vi "initializeRobotModelTest.vi"(4 "V_sample":dbl, 5 "start":bool, 6 "delta":dbl, 7 "V_sent":dbl, 9 "Samples":dbl, 11 "fixed_V_sent?":bool=TRUE) -> (1 "RobotModelAllInformation out":T1={"distance"=0.0, "lastRobotPosition"=[], "timestampOn2ndStateStart"=timestamp(0 s since 1904-01-01), "sampleCount"=0, "stateInMachine"=0, "crashCases"=[], "lastEstVel"=inf, "IdealVelocities"=[], "RealVelocities"=[], "testFinished?"=FALSE, "RobotModelArray"=[]}, 2 "totalNumberOfTests":dbl, 3 "triples (V0, Vf, V_sent)":dbl[][](array[numeric])=[[-6.5, -7.0, -7.0, 0.0], [-6.0, -7.0, -7.0, 1.0], [-5.5, -7.0, -7.0, 2.0], [-5.0, -7.0, -7.0, 3.0], [-4.5, -7.0, -7.0, 4.0], [-4.0, -7.0, -7.0, 5.0], [-3.5, -7.0, -7.0, 6.0], [-3.0, -7.0, -7.0, 7.0], [-2.5, -7.0, -7.0, 8.0], [-2.0, -7.0, -7.0, 9.0], [-1.5, -7.0, -7.0, 10.0], [-1.0, -7.0, -7.0, 11.0], [-0.5, -7.0, -7.0, 12.0], [0.0, -7.0, -7.0, 13.0], [-7.0, -6.5, -6.5, 14.0], [-6.0, -6.5, -6.5, 15.0], [-5.5, -6.5, -6.5, 16.0], [-5.0, -6.5, -6.5, 17.0], [-4.5, -6.5, -6.5, 18.0], [-4.0, -6.5, -6.5, 19.0], [-3.5, -6.5, -6.5, 20.0], [-3.0, -6.5, -6.5, 21.0], [-2.5, -6.5, -6.5, 22.0], [-2.0, -6.5, -6.5, 23.0], [-1.5, -6.5, -6.5, 24.0], [-1.0, -6.5, -6.5, 25.0], [-0.5, -6.5, -6.5, 26.0], [0.0, -6.5, -6.5, 27.0], [-7.0, -6.0, -6.0, 28.0], [-6.5, -6.0, -6.0, 29.0], [-5.5, -6.0, -6.0, 30.0], [-5.0, -6.0, -6.0, 31.0], [-4.5, -6.0, -6.0, 32.0], [-4.0, -6.0, -6.0, 33.0], [-3.5, -6.0, -6.0, 34.0], [-3.0, -6.0, -6.0, 35.0], [-2.5, -6.0, -6.0, 36.0], [-2.0, -6.0, -6.0, 37.0], [-1.5, -6.0, -6.0, 38.0], [-1.0, -6.0, -6.0, 39.0], [-0.5, -6.0, -6.0, 40.0], [0.0, -6.0, -6.0, 41.0], [-7.0, -5.5, -5.5, 42.0], [-6.5, -5.5, -5.5, 43.0], [-6.0, -5.5, -5.5, 44.0], [-5.0, -5.5, -5.5, 45.0], [-4.5, -5.5, -5.5, 46.0], [-4.0, -5.5, -5.5, 47.0], [-3.5, -5.5, -5.5, 48.0], [-3.0, -5.5, -5.5, 49.0], [-2.5, -5.5, -5.5, 50.0], [-2.0, -5.5, -5.5, 51.0], [-1.5, -5.5, -5.5, 52.0], [-1.0, -5.5, -5.5, 53.0], [-0.5, -5.5, -5.5, 54.0], [0.0, -5.5, -5.5, 55.0], [-7.0, -5.0, -5.0, 56.0], [-6.5, -5.0, -5.0, 57.0], [-6.0, -5.0, -5.0, 58.0], [-5.5, -5.0, -5.0, 59.0], [-4.5, -5.0, -5.0, 60.0], [-4.0, -5.0, -5.0, 61.0], [-3.5, -5.0, -5.0, 62.0], [-3.0, -5.0, -5.0, 63.0], [-2.5, -5.0, -5.0, 64.0], [-2.0, -5.0, -5.0, 65.0], [-1.5, -5.0, -5.0, 66.0], [-1.0, -5.0, -5.0, 67.0], [-0.5, -5.0, -5.0, 68.0], [0.0, -5.0, -5.0, 69.0], [-7.0, -4.5, -4.5, 70.0], [-6.5, -4.5, -4.5, 71.0], [-6.0, -4.5, -4.5, 72.0], [-5.5, -4.5, -4.5, 73.0], [-5.0, -4.5, -4.5, 74.0], [-4.0, -4.5, -4.5, 75.0], [-3.5, -4.5, -4.5, 76.0], [-3.0, -4.5, -4.5, 77.0], [-2.5, -4.5, -4.5, 78.0], [-2.0, -4.5, -4.5, 79.0], [-1.5, -4.5, -4.5, 80.0], [-1.0, -4.5, -4.5, 81.0], [-0.5, -4.5, -4.5, 82.0], [0.0, -4.5, -4.5, 83.0], [-7.0, -4.0, -4.0, 84.0], [-6.5, -4.0, -4.0, 85.0], [-6.0, -4.0, -4.0, 86.0], [-5.5, -4.0, -4.0, 87.0], [-5.0, -4.0, -4.0, 88.0], [-4.5, -4.0, -4.0, 89.0], [-3.5, -4.0, -4.0, 90.0], [-3.0, -4.0, -4.0, 91.0], [-2.5, -4.0, -4.0, 92.0], [-2.0, -4.0, -4.0, 93.0], [-1.5, -4.0, -4.0, 94.0], [-1.0, -4.0, -4.0, 95.0], [-0.5, -4.0, -4.0, 96.0], [0.0, -4.0, -4.0, 97.0], [-7.0, -3.5, -3.5, 98.0], [-6.5, -3.5, -3.5, 99.0], [-6.0, -3.5, -3.5, 100.0], [-5.5, -3.5, -3.5, 101.0], [-5.0, -3.5, -3.5, 102.0], [-4.5, -3.5, -3.5, 103.0], [-4.0, -3.5, -3.5, 104.0], [-3.0, -3.5, -3.5, 105.0], [-2.5, -3.5, -3.5, 106.0], [-2.0, -3.5, -3.5, 107.0], [-1.5, -3.5, -3.5, 108.0], [-1.0, -3.5, -3.5, 109.0], [-0.5, -3.5, -3.5, 110.0], [0.0, -3.5, -3.5, 111.0], [-7.0, -3.0, -3.0, 112.0], [-6.5, -3.0, -3.0, 113.0], [-6.0, -3.0, -3.0, 114.0], [-5.5, -3.0, -3.0, 115.0], [-5.0, -3.0, -3.0, 116.0], [-4.5, -3.0, -3.0, 117.0], [-4.0, -3.0, -3.0, 118.0], [-3.5, -3.0, -3.0, 119.0], [-2.5, -3.0, -3.0, 120.0], [-2.0, -3.0, -3.0, 121.0], [-1.5, -3.0, -3.0, 122.0], [-1.0, -3.0, -3.0, 123.0], [-0.5, -3.0, -3.0, 124.0], [0.0, -3.0, -3.0, 125.0], [-7.0, -2.5, -2.5, 126.0], [-6.5, -2.5, -2.5, 127.0], [-6.0, -2.5, -2.5, 128.0], [-5.5, -2.5, -2.5, 129.0], [-5.0, -2.5, -2.5, 130.0], [-4.5, -2.5, -2.5, 131.0], [-4.0, -2.5, -2.5, 132.0], [-3.5, -2.5, -2.5, 133.0], [-3.0, -2.5, -2.5, 134.0], [-2.0, -2.5, -2.5, 135.0], [-1.5, -2.5, -2.5, 136.0], [-1.0, -2.5, -2.5, 137.0], [-0.5, -2.5, -2.5, 138.0], [0.0, -2.5, -2.5, 139.0], [-7.0, -2.0, -2.0, 140.0], [-6.5, -2.0, -2.0, 141.0], [-6.0, -2.0, -2.0, 142.0], [-5.5, -2.0, -2.0, 143.0], [-5.0, -2.0, -2.0, 144.0], [-4.5, -2.0, -2.0, 145.0], [-4.0, -2.0, -2.0, 146.0], [-3.5, -2.0, -2.0, 147.0], [-3.0, -2.0, -2.0, 148.0], [-2.5, -2.0, -2.0, 149.0], [-1.5, -2.0, -2.0, 150.0], [-1.0, -2.0, -2.0, 151.0], [-0.5, -2.0, -2.0, 152.0], [0.0, -2.0, -2.0, 153.0], [-7.0, -1.5, -1.5, 154.0], [-6.5, -1.5, -1.5, 155.0], [-6.0, -1.5, -1.5, 156.0], [-5.5, -1.5, -1.5, 157.0], [-5.0, -1.5, -1.5, 158.0], [-4.5, -1.5, -1.5, 159.0], [-4.0, -1.5, -1.5, 160.0], [-3.5, -1.5, -1.5, 161.0], [-3.0, -1.5, -1.5, 162.0], [-2.5, -1.5, -1.5, 163.0], [-2.0, -1.5, -1.5, 164.0], [-1.0, -1.5, -1.5, 165.0], [-0.5, -1.5, -1.5, 166.0], [0.0, -1.5, -1.5, 167.0], [-7.0, -1.0, -1.0, 168.0], [-6.5, -1.0, -1.0, 169.0], [-6.0, -1.0, -1.0, 170.0], [-5.5, -1.0, -1.0, 171.0], [-5.0, -1.0, -1.0, 172.0], [-4.5, -1.0, -1.0, 173.0], [-4.0, -1.0, -1.0, 174.0], [-3.5, -1.0, -1.0, 175.0], [-3.0, -1.0, -1.0, 176.0], [-2.5, -1.0, -1.0, 177.0], [-2.0, -1.0, -1.0, 178.0], [-1.5, -1.0, -1.0, 179.0], [-0.5, -1.0, -1.0, 180.0], [0.0, -1.0, -1.0, 181.0], [-7.0, -0.5, -0.5, 182.0], [-6.5, -0.5, -0.5, 183.0], [-6.0, -0.5, -0.5, 184.0], [-5.5, -0.5, -0.5, 185.0], [-5.0, -0.5, -0.5, 186.0], [-4.5, -0.5, -0.5, 187.0], [-4.0, -0.5, -0.5, 188.0], [-3.5, -0.5, -0.5, 189.0], [-3.0, -0.5, -0.5, 190.0], [-2.5, -0.5, -0.5, 191.0], [-2.0, -0.5, -0.5, 192.0], [-1.5, -0.5, -0.5, 193.0], [-1.0, -0.5, -0.5, 194.0], [0.0, -0.5, -0.5, 195.0], [-7.0, 0.0, 0.0, 196.0], [-6.5, 0.0, 0.0, 197.0], [-6.0, 0.0, 0.0, 198.0], [-5.5, 0.0, 0.0, 199.0], [-5.0, 0.0, 0.0, 200.0], [-4.5, 0.0, 0.0, 201.0], [-4.0, 0.0, 0.0, 202.0], [-3.5, 0.0, 0.0, 203.0], [-3.0, 0.0, 0.0, 204.0], [-2.5, 0.0, 0.0, 205.0], [-2.0, 0.0, 0.0, 206.0], [-1.5, 0.0, 0.0, 207.0], [-1.0, 0.0, 0.0, 208.0], [-0.5, 0.0, 0.0, 209.0], [0.5, 0.0, 0.0, 210.0], [1.0, 0.0, 0.0, 211.0], [1.5, 0.0, 0.0, 212.0], [2.0, 0.0, 0.0, 213.0], [2.5, 0.0, 0.0, 214.0], [3.0, 0.0, 0.0, 215.0], [3.5, 0.0, 0.0, 216.0], [4.0, 0.0, 0.0, 217.0], [4.5, 0.0, 0.0, 218.0], [5.0, 0.0, 0.0, 219.0], [5.5, 0.0, 0.0, 220.0], [6.0, 0.0, 0.0, 221.0], [6.5, 0.0, 0.0, 222.0], [7.0, 0.0, 0.0, 223.0], [0.0, 0.5, 0.5, 224.0], [1.0, 0.5, 0.5, 225.0], [1.5, 0.5, 0.5, 226.0], [2.0, 0.5, 0.5, 227.0], [2.5, 0.5, 0.5, 228.0], [3.0, 0.5, 0.5, 229.0], [3.5, 0.5, 0.5, 230.0], [4.0, 0.5, 0.5, 231.0], [4.5, 0.5, 0.5, 232.0], [5.0, 0.5, 0.5, 233.0], [5.5, 0.5, 0.5, 234.0], [6.0, 0.5, 0.5, 235.0], [6.5, 0.5, 0.5, 236.0], [7.0, 0.5, 0.5, 237.0], [0.0, 1.0, 1.0, 238.0], [0.5, 1.0, 1.0, 239.0], [1.5, 1.0, 1.0, 240.0], [2.0, 1.0, 1.0, 241.0], [2.5, 1.0, 1.0, 242.0], [3.0, 1.0, 1.0, 243.0], [3.5, 1.0, 1.0, 244.0], [4.0, 1.0, 1.0, 245.0], [4.5, 1.0, 1.0, 246.0], [5.0, 1.0, 1.0, 247.0], [5.5, 1.0, 1.0, 248.0], [6.0, 1.0, 1.0, 249.0], [6.5, 1.0, 1.0, 250.0], [7.0, 1.0, 1.0, 251.0], [0.0, 1.5, 1.5, 252.0], [0.5, 1.5, 1.5, 253.0], [1.0, 1.5, 1.5, 254.0], [2.0, 1.5, 1.5, 255.0], [2.5, 1.5, 1.5, 256.0], [3.0, 1.5, 1.5, 257.0], [3.5, 1.5, 1.5, 258.0], [4.0, 1.5, 1.5, 259.0], [4.5, 1.5, 1.5, 260.0], [5.0, 1.5, 1.5, 261.0], [5.5, 1.5, 1.5, 262.0], [6.0, 1.5, 1.5, 263.0], [6.5, 1.5, 1.5, 264.0], [7.0, 1.5, 1.5, 265.0], [0.0, 2.0, 2.0, 266.0], [0.5, 2.0, 2.0, 267.0], [1.0, 2.0, 2.0, 268.0], [1.5, 2.0, 2.0, 269.0], [2.5, 2.0, 2.0, 270.0], [3.0, 2.0, 2.0, 271.0], [3.5, 2.0, 2.0, 272.0], [4.0, 2.0, 2.0, 273.0], [4.5, 2.0, 2.0, 274.0], [5.0, 2.0, 2.0, 275.0], [5.5, 2.0, 2.0, 276.0], [6.0, 2.0, 2.0, 277.0], [6.5, 2.0, 2.0, 278.0], [7.0, 2.0, 2.0, 279.0], [0.0, 2.5, 2.5, 280.0], [0.5, 2.5, 2.5, 281.0], [1.0, 2.5, 2.5, 282.0], [1.5, 2.5, 2.5, 283.0], [2.0, 2.5, 2.5, 284.0], [3.0, 2.5, 2.5, 285.0], [3.5, 2.5, 2.5, 286.0], [4.0, 2.5, 2.5, 287.0], [4.5, 2.5, 2.5, 288.0], [5.0, 2.5, 2.5, 289.0], [5.5, 2.5, 2.5, 290.0], [6.0, 2.5, 2.5, 291.0], [6.5, 2.5, 2.5, 292.0], [7.0, 2.5, 2.5, 293.0], [0.0, 3.0, 3.0, 294.0], [0.5, 3.0, 3.0, 295.0], [1.0, 3.0, 3.0, 296.0], [1.5, 3.0, 3.0, 297.0], [2.0, 3.0, 3.0, 298.0], [2.5, 3.0, 3.0, 299.0], [3.5, 3.0, 3.0, 300.0], [4.0, 3.0, 3.0, 301.0], [4.5, 3.0, 3.0, 302.0], [5.0, 3.0, 3.0, 303.0], [5.5, 3.0, 3.0, 304.0], [6.0, 3.0, 3.0, 305.0], [6.5, 3.0, 3.0, 306.0], [7.0, 3.0, 3.0, 307.0], [0.0, 3.5, 3.5, 308.0], [0.5, 3.5, 3.5, 309.0], [1.0, 3.5, 3.5, 310.0], [1.5, 3.5, 3.5, 311.0], [2.0, 3.5, 3.5, 312.0], [2.5, 3.5, 3.5, 313.0], [3.0, 3.5, 3.5, 314.0], [4.0, 3.5, 3.5, 315.0], [4.5, 3.5, 3.5, 316.0], [5.0, 3.5, 3.5, 317.0], [5.5, 3.5, 3.5, 318.0], [6.0, 3.5, 3.5, 319.0], [6.5, 3.5, 3.5, 320.0], [7.0, 3.5, 3.5, 321.0], [0.0, 4.0, 4.0, 322.0], [0.5, 4.0, 4.0, 323.0], [1.0, 4.0, 4.0, 324.0], [1.5, 4.0, 4.0, 325.0], [2.0, 4.0, 4.0, 326.0], [2.5, 4.0, 4.0, 327.0], [3.0, 4.0, 4.0, 328.0], [3.5, 4.0, 4.0, 329.0], [4.5, 4.0, 4.0, 330.0], [5.0, 4.0, 4.0, 331.0], [5.5, 4.0, 4.0, 332.0], [6.0, 4.0, 4.0, 333.0], [6.5, 4.0, 4.0, 334.0], [7.0, 4.0, 4.0, 335.0], [0.0, 4.5, 4.5, 336.0], [0.5, 4.5, 4.5, 337.0], [1.0, 4.5, 4.5, 338.0], [1.5, 4.5, 4.5, 339.0], [2.0, 4.5, 4.5, 340.0], [2.5, 4.5, 4.5, 341.0], [3.0, 4.5, 4.5, 342.0], [3.5, 4.5, 4.5, 343.0], [4.0, 4.5, 4.5, 344.0], [5.0, 4.5, 4.5, 345.0], [5.5, 4.5, 4.5, 346.0], [6.0, 4.5, 4.5, 347.0], [6.5, 4.5, 4.5, 348.0], [7.0, 4.5, 4.5, 349.0], [0.0, 5.0, 5.0, 350.0], [0.5, 5.0, 5.0, 351.0], [1.0, 5.0, 5.0, 352.0], [1.5, 5.0, 5.0, 353.0], [2.0, 5.0, 5.0, 354.0], [2.5, 5.0, 5.0, 355.0], [3.0, 5.0, 5.0, 356.0], [3.5, 5.0, 5.0, 357.0], [4.0, 5.0, 5.0, 358.0], [4.5, 5.0, 5.0, 359.0], [5.5, 5.0, 5.0, 360.0], [6.0, 5.0, 5.0, 361.0], [6.5, 5.0, 5.0, 362.0], [7.0, 5.0, 5.0, 363.0], [0.0, 5.5, 5.5, 364.0], [0.5, 5.5, 5.5, 365.0], [1.0, 5.5, 5.5, 366.0], [1.5, 5.5, 5.5, 367.0], [2.0, 5.5, 5.5, 368.0], [2.5, 5.5, 5.5, 369.0], [3.0, 5.5, 5.5, 370.0], [3.5, 5.5, 5.5, 371.0], [4.0, 5.5, 5.5, 372.0], [4.5, 5.5, 5.5, 373.0], [5.0, 5.5, 5.5, 374.0], [6.0, 5.5, 5.5, 375.0], [6.5, 5.5, 5.5, 376.0], [7.0, 5.5, 5.5, 377.0], [0.0, 6.0, 6.0, 378.0], [0.5, 6.0, 6.0, 379.0], [1.0, 6.0, 6.0, 380.0], [1.5, 6.0, 6.0, 381.0], [2.0, 6.0, 6.0, 382.0], [2.5, 6.0, 6.0, 383.0], [3.0, 6.0, 6.0, 384.0], [3.5, 6.0, 6.0, 385.0], [4.0, 6.0, 6.0, 386.0], [4.5, 6.0, 6.0, 387.0], [5.0, 6.0, 6.0, 388.0], [5.5, 6.0, 6.0, 389.0], [6.5, 6.0, 6.0, 390.0], [7.0, 6.0, 6.0, 391.0], [0.0, 6.5, 6.5, 392.0], [0.5, 6.5, 6.5, 393.0], [1.0, 6.5, 6.5, 394.0], [1.5, 6.5, 6.5, 395.0], [2.0, 6.5, 6.5, 396.0], [2.5, 6.5, 6.5, 397.0], [3.0, 6.5, 6.5, 398.0], [3.5, 6.5, 6.5, 399.0], [4.0, 6.5, 6.5, 400.0], [4.5, 6.5, 6.5, 401.0], [5.0, 6.5, 6.5, 402.0], [5.5, 6.5, 6.5, 403.0], [6.0, 6.5, 6.5, 404.0], [7.0, 6.5, 6.5, 405.0], [0.0, 7.0, 7.0, 406.0], [0.5, 7.0, 7.0, 407.0], [1.0, 7.0, 7.0, 408.0], [1.5, 7.0, 7.0, 409.0], [2.0, 7.0, 7.0, 410.0], [2.5, 7.0, 7.0, 411.0], [3.0, 7.0, 7.0, 412.0], [3.5, 7.0, 7.0, 413.0], [4.0, 7.0, 7.0, 414.0], [4.5, 7.0, 7.0, 415.0], [5.0, 7.0, 7.0, 416.0], [5.5, 7.0, 7.0, 417.0], [6.0, 7.0, 7.0, 418.0], [6.5, 7.0, 7.0, 419.0]])   [LabVIEW 2021, in "Game.lvclass"]
uses:
  Game.lvclass
  Controls/RobotModelAllInformation.ctl
  Controls/RobotModelTestCrashCase.ctl
  VelocityPlanningTest/Controls/robotModelArray.ctl
  Controls/RobotModel.ctl
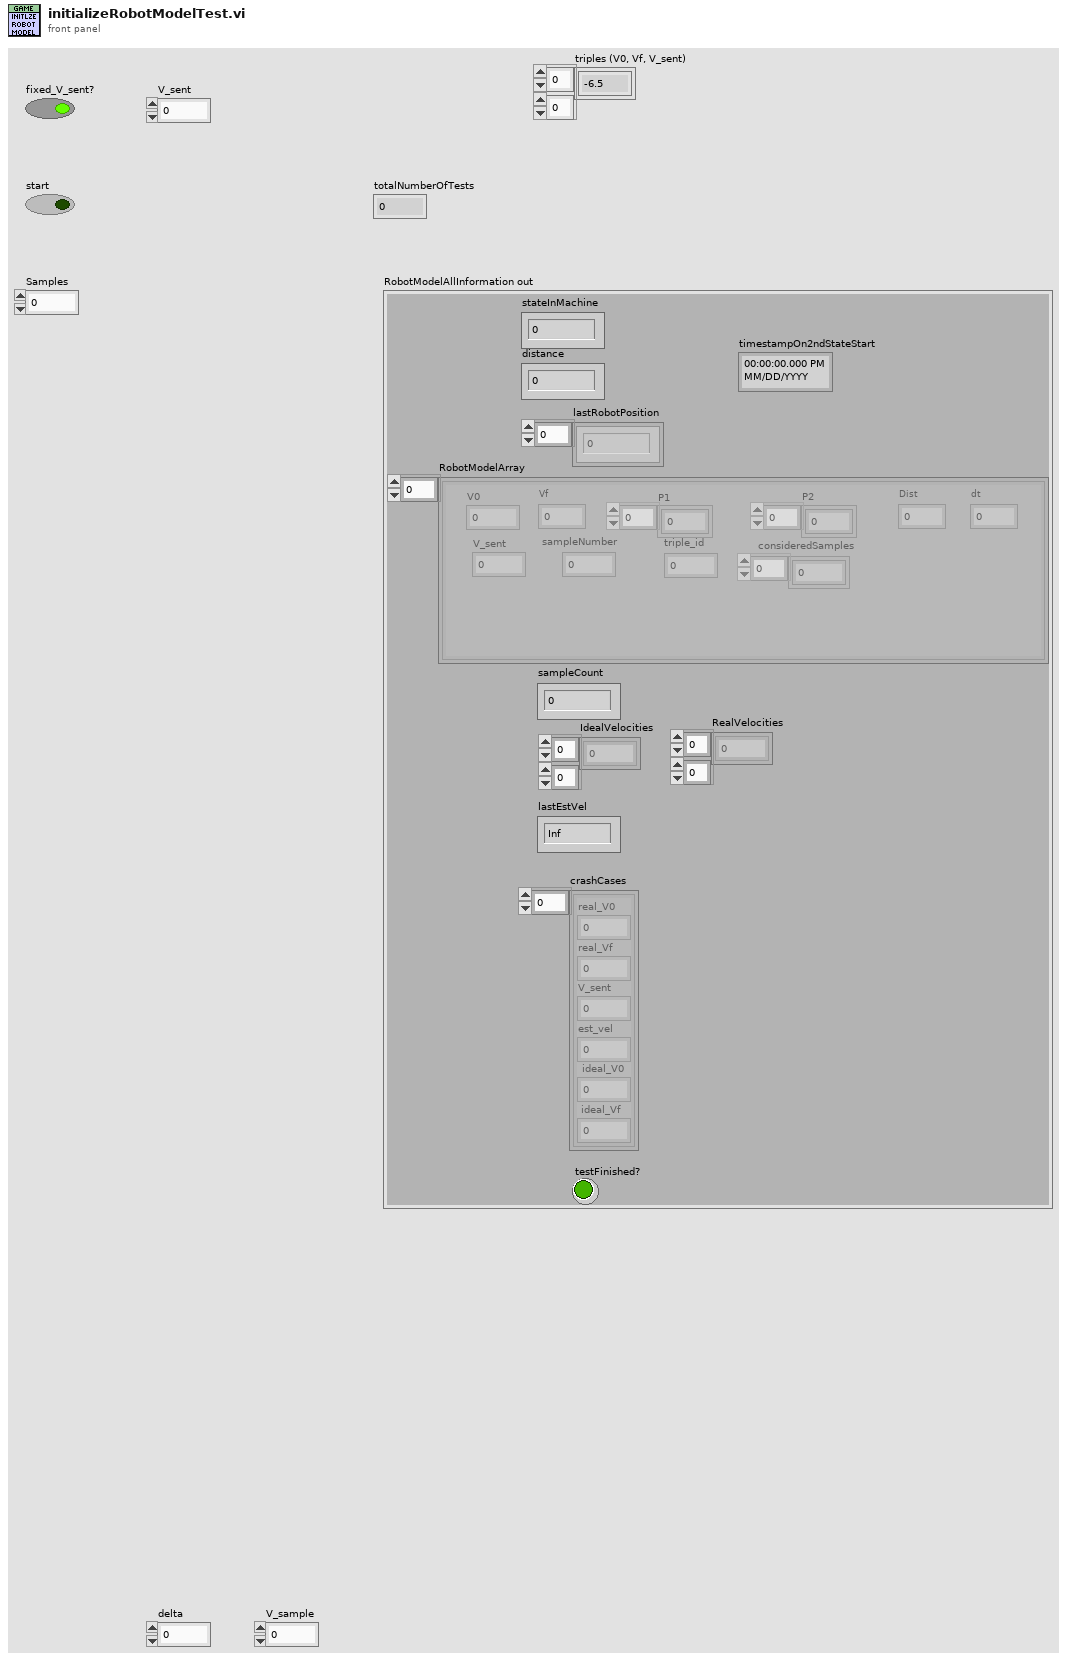
[diagram p1: front panel]
types:
  T1 = typedef "RobotModelAllInformation.ctl" = cluster{"distance":dbl, "lastRobotPosition":dbl[], "timestampOn2ndStateStart":timestamp, "sampleCount":i32, "stateInMachine":i32, "crashCases":T2[], "lastEstVel":dbl, "IdealVelocities":dbl[][], "RealVelocities":dbl[][], "testFinished?":bool, "RobotModelArray":T3}
  T2 = typedef "RobotModelTestCrashCase.ctl" = cluster{"real_V0":dbl, "real_Vf":dbl, "V_sent":dbl, "est_vel":dbl, "ideal_V0":dbl, "ideal_Vf":dbl}
  T3 = typedef "robotModelArray.ctl" = T4[]
  T4 = typedef "RobotModel.ctl" = cluster{"V0":dbl, "Vf":dbl, "Dist":dbl, "dt":dbl, "P1":dbl[], "P2":dbl[], "V_sent":dbl, "sampleNumber":i32, "triple_id":i32, "consideredSamples":dbl[]}
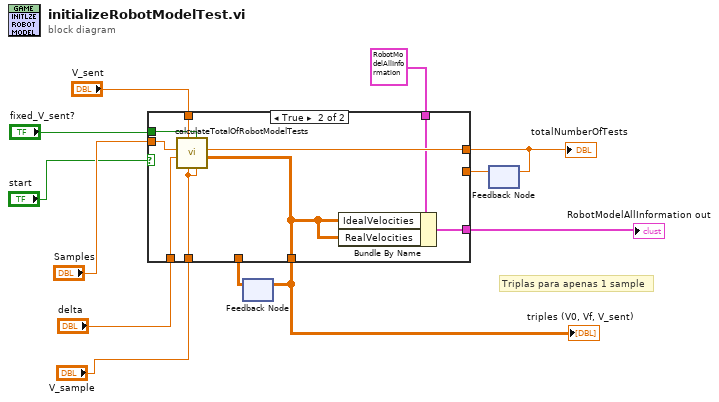
[diagram p0: block diagram]
diagram:
  # "Triplas para apenas 1 sample"
  n1 = feedback #1() -> (w1:dbl[][])  [unwired: 1 in]
  n2 = feedback #2() -> (w5:dbl)  [unwired: 1 in]
  n3 = case shown="True" "start" {
    tunnel: [w15 w24] -> w4
    tunnel: "Samples" -> [_ w23]
    tunnel: "delta" -> [_ w22]
    tunnel: "V_sample" -> [_ w21]
    tunnel: "V_sent" -> [_ w20]
    tunnel: w5 -> [w15 _]
    tunnel: "fixed_V_sent?" -> [_ w19]
    tunnel: T1 {"distance"=0.0, "lastRobotPosition"=[], "timestampOn2ndStateStart"=timestamp(0 s since 1904-01-01), "sampleCount"=0, "stateInMachine"=0, "crashCases"=[], "lastEstVel"=inf, "IdealVelocities"=[], "RealVelocities"=[], "testFinished?"=FALSE, "RobotModelArray"=[]} ("RobotModelAllInformation in") -> [w14 w18]
    tunnel: [w14 w17] -> w12
    tunnel: [w13 w16] -> w2
    tunnel: w1 -> [w13 _]
    frame False {
    }
    frame True {
      n4 = call "calculateTotalOfRobotModelTests.vi"("Vf"=w21, "fixed_V_sent?"=w19, "V0"=w21, "V_sent"=w20, "delta"=w22, "quantity of samples"=w23) -> ("triples (V0, Vf, V_sent)"=w16:dbl[][], "totalNumerOfTests"=w24:dbl)  [unwired: 2 in, 2 out]
      n5 = Bundle By Name(cluster=w18, "IdealVelocities"=w16, "RealVelocities"=w16) -> (w17:T1)
    }
  }
  "RobotModelAllInformation out" <- w12
  "totalNumberOfTests" <- w4
  "triples (V0, Vf, V_sent)" <- w2
  n6 = feedback-in #1(w2) -> ()
  n7 = feedback-in #2(w4) -> ()
